vi "SDCP SMF Receiver and Transmitter - Test with plot.vi"() -> ()   [LabVIEW 2020]
uses:
  Typedefs/SDCP - Serial Port Control - Commands.ctl
  Typedefs/SDCP - Standard Message Frame Parameters - FGV - commands.ctl
  <vilib>/Utility/miscctls.llb/LVComboBoxStrsAndValuesArrayTypeDef.ctl
panel:
  in  "Remove frame":bool
  in  "Frame to add":string(combo)
  in  "Add frame":bool
  in  "Transmit Table":string[][](table)
  out "Elapsed time (ms)":u32
  in  "Parameter file path":path
  in  "Receive Table":i32(listbox)
  in  "stop":bool
  in  "VISA resource name":refnum<visa-resource-name>
  in  "Baud rate":u32=9600
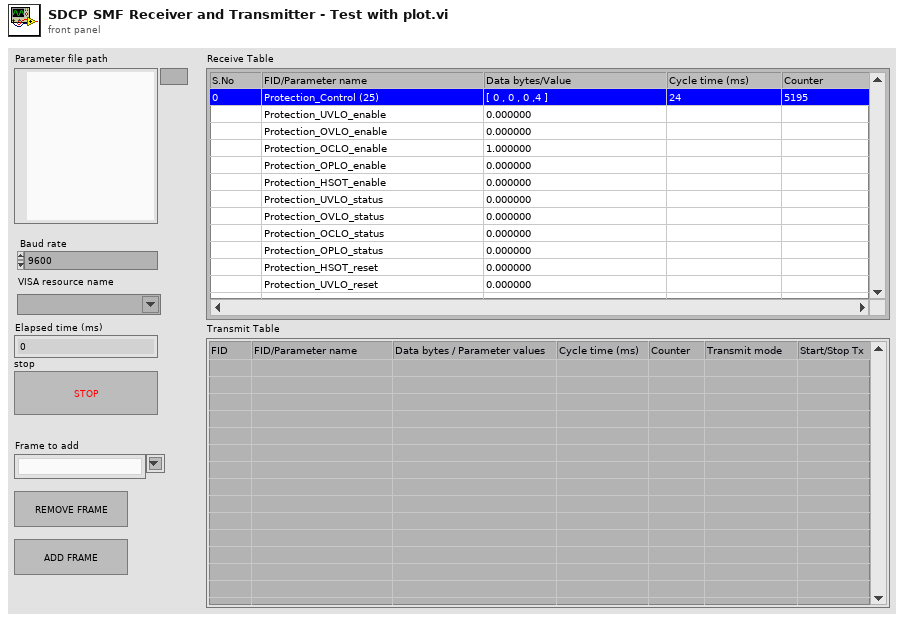
[diagram p1: front panel]
types:
  T1 = enum16{"Initialize", "Add row", "Remove row", "Update"}
  T2 = typedef "LVComboBoxStrsAndValuesArrayTypeDef.ctl" = cluster{"String":string, "Value":string}[]
  T3 = typedef "SDCP - Standard Message Frame Parameters - FGV - commands.ctl" = enum16{"Write descriptors", "Read descriptors", "Read values", "Load parameters from file", "Write values"}
  T4 = typedef "SDCP - Serial Port Control - Commands.ctl" = enum16{"Open", "Read", "Write", "Get instance", "Close"}
  T5 = typedef "SDCP - SMF parameter descriptors.ctl" = cluster{"Frame name":string, "Frame ID":i32, "Data type":string, "Start Position":i32, "Length":i32, "Factor":dbl, "Offset":dbl, "Parameter name":string, "Value":string}
  T6 = typedef "SDCP SMF Receiver and Transmitter - Notifier and Queues.ctl" = cluster{"Trace Queue":refnum<queue>, "Tx - Log Table Queue":refnum<queue>, "Tx - User Queue":refnum<queue>, "Rx - Log Table Queue":refnum<queue>, "Rx - User Queue":refnum<queue>, "Log status Notifier":refnum<notifier>, "Plot Queue":refnum<queue>}
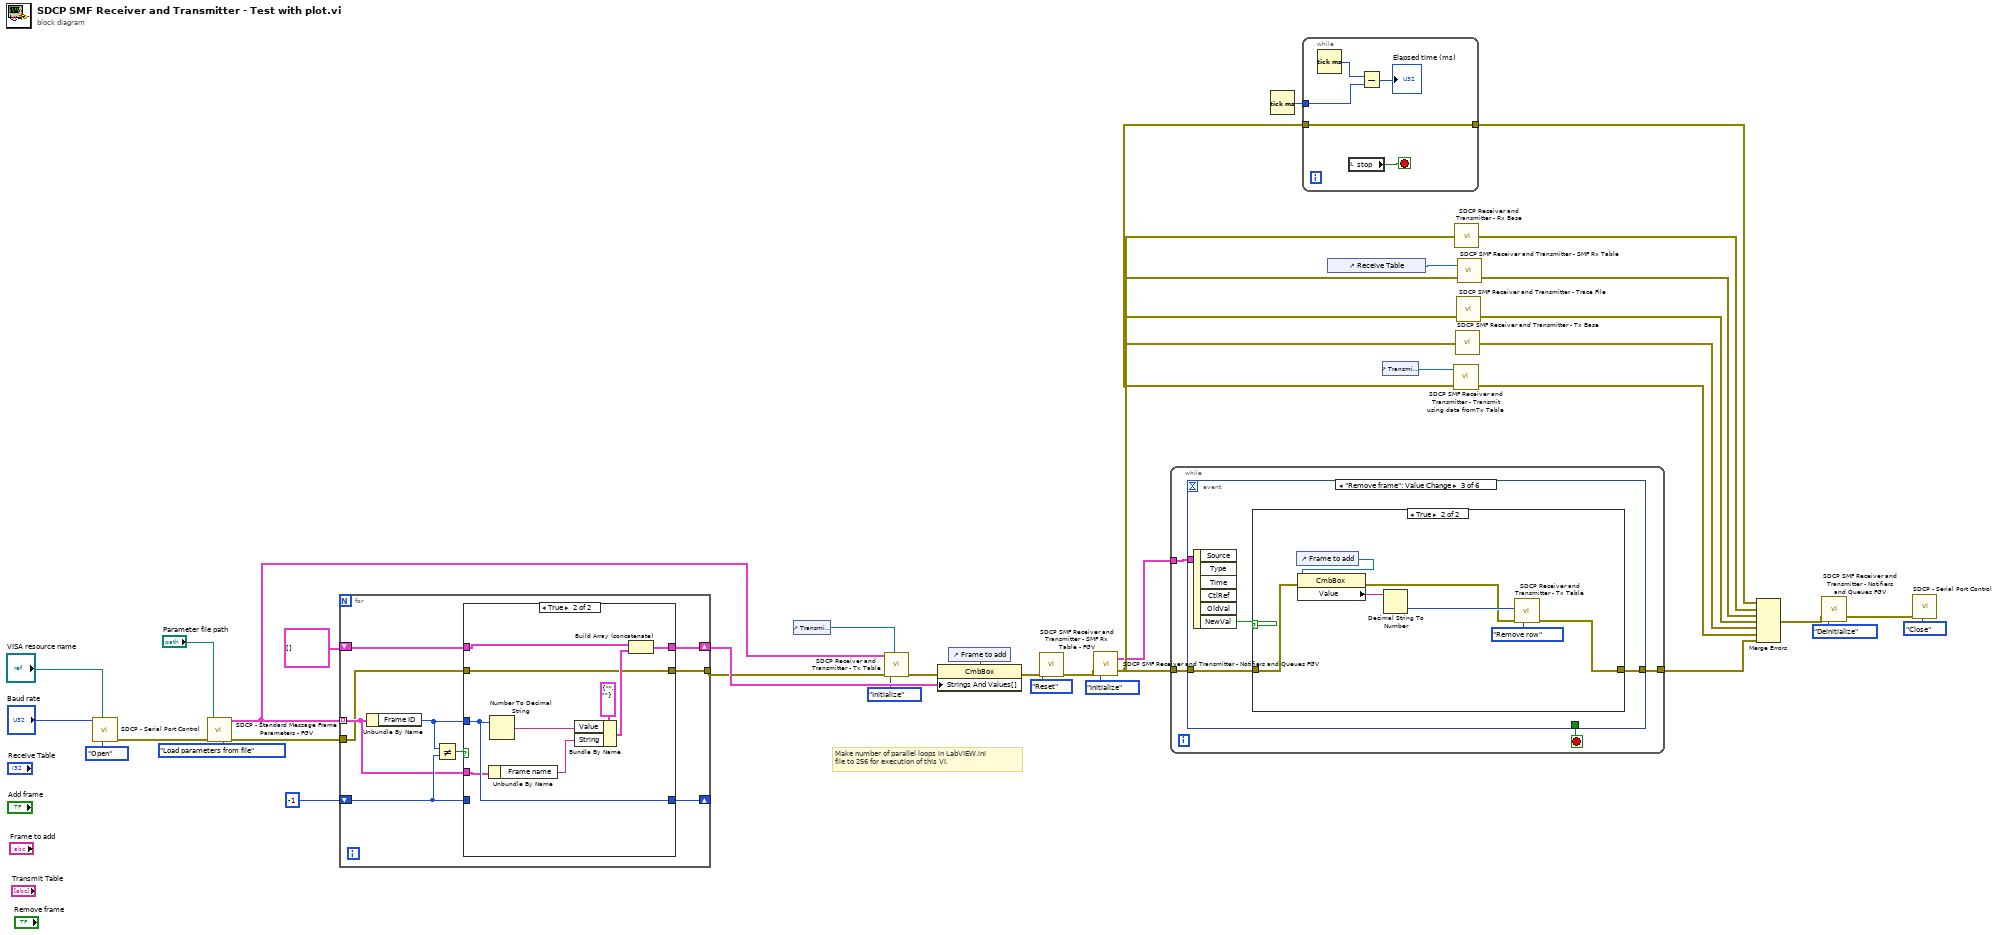
[diagram p0: block diagram]
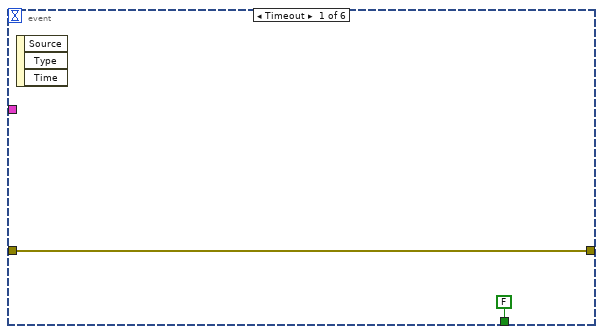
[diagram p2: hidden frame]
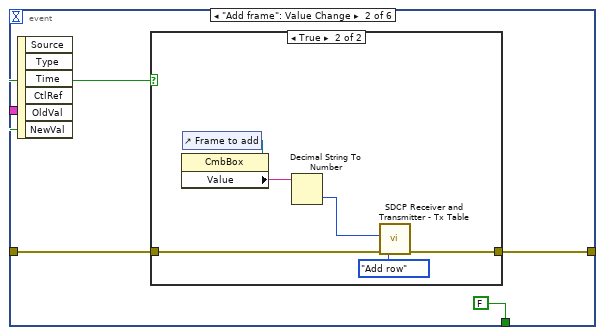
[diagram p3: hidden frame]
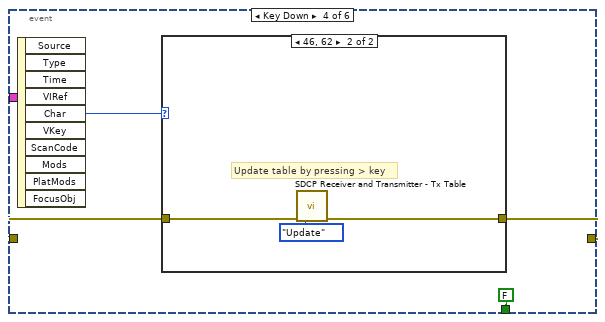
[diagram p6: hidden frame]
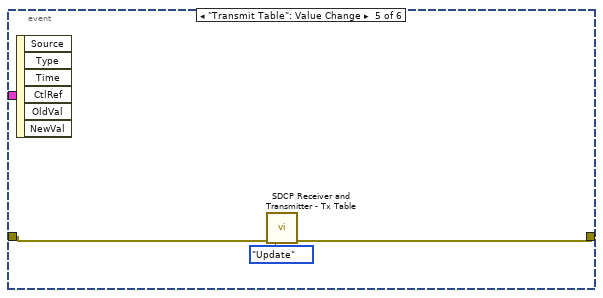
[diagram p8: hidden frame]
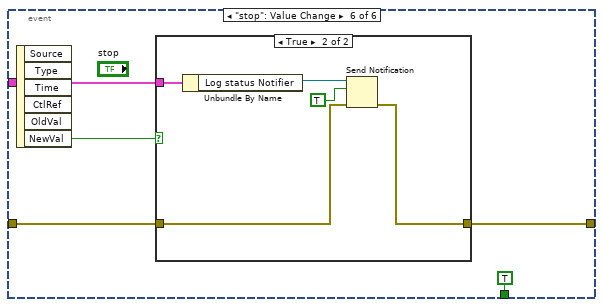
[diagram p9: hidden frame]
diagram:
  # "Make number of parallel loops in LabVIEW.ini\nfile to 256 for execution of this VI."
  n1 = call "SDCP - Serial Port Control.vi"("Command"=SDCP_-_Serial_Port_Control_-_Commands."Open", "VISA resource name"="VISA resource name", "Baud rate"="Baud rate") -> ("error out"=w22:errorcluster)  [unwired: 6 in, 2 out]
  n2 = call "SDCP - Standard Message Frame Parameters - FGV.vi"("Parameter file path"="Parameter file path", "error in (no error)"=w22, "Command"=SDCP_-_Standard_Message_Frame_Parameters_-_FGV_-_commands."Load parameters from file") -> ("SMF Parameters descriptors out"=w12:T5[], "error out"=w18:errorcluster)  [unwired: 4 in]
  n3 = for {
    tunnel: w18 -> [w38]
    tunnel: w12 -> [w39] mode=indexing
    shift-right: [w43] -> _
    shift-left: -1 -> [w42]
    shift-right: [w40] -> w14
    shift-left: T2 [] ("Strings And Values []") -> [w41]
    tunnel: [w37] -> w13
    n4 = Unbundle By Name(w39) -> ("Frame ID"=w44:i32)
    n5 = Not Equal?(x=w44, y=w42) -> (x != y?=w45:bool)
    n6 = case shown="True" w45 {
      tunnel: w44 -> [_ w57]
      tunnel: [w48 w57] -> w43
      tunnel: w42 -> [w48 _]
      tunnel: w41 -> [w47 w52]
      tunnel: [w47 w50] -> w40
      tunnel: w39 -> [_ w54]
      tunnel: w38 -> [w46 w49]
      tunnel: [w46 w49] -> w37
      frame False {
      }
      frame True {
        n7 = Unbundle By Name(w54) -> ("Frame name"=w53:string)
        n8 = Number To Decimal String(number=w57) -> (decimal integer string=w55:string)  [unwired: 1 in]
        n9 = Bundle By Name(cluster=cluster{"String":string, "Value":string} {"String"="", "Value"=""}, "Value"=w55, "String"=w53) -> (w51:cluster{"String":string, "Value":string})
        n10 = Build Array (concatenate)(w52, w51) -> (w50:T2)
      }
    }
  }
  n11 = control-ref of="Transmit Table"() -> (w9:refnum<vi>)
  n12 = call "SDCP Receiver and Transmitter - Tx Table.vi"("Table Control"=w9, "error in (no error)"=w13, "Command"=T1."Initialize", "SMF Parameters descriptors"=w12) -> ("error out"=w7:errorcluster)  [unwired: 6 in, 1 out]
  n13 = control-ref of="Frame to add"() -> (w8:refnum<vi>)
  n14 = property class="CmbBox"(reference=w8, error in=w7, "Strings And Values[]"=w14) -> (error out=w15:errorcluster)  [unwired: 1 out]
  n15 = call "SDCP SMF Receiver and Transmitter - SMF Rx Table - FGV.vi"("error in (no error)"=w15, "Command"=enum16{"Reset", "Write", "Read"}."Reset") -> ("error out"=w29:errorcluster)  [unwired: 8 in, 1 out]
  n16 = call "SDCP SMF Receiver and Transmitter - Notifiers and Queues FGV.vi"("error in (no error)"=w29, "Command"=enum16{"Initialize", "Read", "Deinitialize"}."Initialize") -> ("error out"=w5:errorcluster, "Output"=w1:T6)
  n17 = while {
    tunnel: w5 -> [w61]
    tunnel: [w60] -> w2
    tunnel: w1 -> [w58]
    stop <- w59 stop-if-true
    n18 = event shown="[2] \"Remove frame\": Value Change" {
      selector: _ -> [_ _ _ _ _ _]
      dyn-events: _ -> [_ _ _ _ _ _]
      timeout: _ -> [_ _ _ _ _ _]
      tunnel: w61 -> [w63 w66 w77 w88 w95 w98]
      tunnel: [w63 w65 w76 w87 w94 w97] -> w60
      tunnel: [FALSE FALSE _ FALSE _ TRUE] -> w59
      tunnel: w58 -> [_ _ _ _ _ w100]
      event Timeout {
        n19 = event-data() -> ()  [unwired: 1 in, 3 out]
      }
      event "Add frame": Value Change {
        n20 = event-data() -> ("NewVal"=w67:bool)  [unwired: 1 in, 5 out]
        n21 = case shown="True" w67 {
          tunnel: w66 -> [w68 w72]
          tunnel: [w68 w70] -> w65
          frame False {
          }
          frame True {
            n22 = control-ref of="Frame to add"() -> (w74:refnum<vi>)
            n23 = property class="CmbBox"(reference=w74) -> ("Value"=w73:string)  [unwired: 1 in, 2 out]
            n24 = Decimal String To Number(string=w73) -> (number=w71:i32)  [unwired: 2 in, 1 out]
            n25 = call "SDCP Receiver and Transmitter - Tx Table.vi"("error in (no error)"=w72, "Command"=T1."Add row", "FID"=w71) -> ("error out"=w70:errorcluster)  [unwired: 7 in, 1 out]
          }
        }
      }
      event "Remove frame": Value Change {
        n26 = event-data() -> ("NewVal"=w75:bool)  [unwired: 1 in, 5 out]
        n27 = case shown="True" w75 {
          tunnel: w77 -> [w78 w83]
          tunnel: [w78 w80] -> w76
          frame False {
          }
          frame True {
            n28 = control-ref of="Frame to add"() -> (w82:refnum<vi>)
            n29 = property class="CmbBox"(reference=w82, error in=w83) -> (error out=w81:errorcluster, "Value"=w85:string)  [unwired: 1 out]
            n30 = Decimal String To Number(string=w85) -> (number=w84:i32)  [unwired: 2 in, 1 out]
            n31 = call "SDCP Receiver and Transmitter - Tx Table.vi"("error in (no error)"=w81, "Command"=T1."Remove row", "FID"=w84) -> ("error out"=w80:errorcluster)  [unwired: 7 in, 1 out]
          }
        }
      }
      event Key Down {
        n32 = event-data() -> ("Char"=w86:i16)  [unwired: 1 in, 9 out]
        n33 = case shown="46, 62" w86 {
          tunnel: w88 -> [w90 w92]
          tunnel: [w90 w91] -> w87
          frame 0, Default {
          }
          frame 46, 62 {
            # "Update table by pressing > key"
            n34 = call "SDCP Receiver and Transmitter - Tx Table.vi"("error in (no error)"=w92, "Command"=T1."Update") -> ("error out"=w91:errorcluster)  [unwired: 8 in, 1 out]
          }
        }
      }
      event "Transmit Table": Value Change {
        n35 = event-data() -> ()  [unwired: 1 in, 6 out]
        n36 = call "SDCP Receiver and Transmitter - Tx Table.vi"("error in (no error)"=w95, "Command"=T1."Update") -> ("error out"=w94:errorcluster)  [unwired: 8 in, 1 out]
      }
      event "stop": Value Change {
        n37 = event-data() -> ("NewVal"=w99:bool)  [unwired: 1 in, 5 out]
        n38 = case shown="True" w99 {
          tunnel: w100 -> [_ w107]
          tunnel: w98 -> [w102 w104]
          tunnel: [w102 w103] -> w97
          frame False {
          }
          frame True {
            n39 = Unbundle By Name(w107) -> ("Log status Notifier"=w106:refnum<notifier>)
            n40 = Send Notification(notification=TRUE, notifier=w106, error in (no error)=w104) -> (error out=w103:errorcluster)  [unwired: 1 out]
          }
        }
      }
    }
  }
  n41 = Tick Count (ms)() -> (millisecond timer value=w19:u32)
  n42 = while {
    tunnel: w5 -> [w111]
    tunnel: [w111] -> w20
    tunnel: w19 -> [w109]
    stop <- w112 stop-if-true
    n43 = Tick Count (ms)() -> (millisecond timer value=w110:u32)
    n44 = local read "stop"() -> (w112:bool)
    n45 = Subtract(x=w110, y=w109) -> (x-y=→"Elapsed time (ms)":u32)
  }
  n46 = control-ref of="Receive Table"() -> (w27:refnum<vi>)
  n47 = control-ref of="Transmit Table"() -> (w6:refnum<vi>)
  n48 = call "SDCP SMF Receiver and Transmitter - Transmit using data fromTx Table.vi"("error in (no error)"=w5, "Table Control"=w6) -> ("error out"=w3:errorcluster)  [unwired: 3 in]
  n49 = call "SDCP Receiver and Transmitter - Rx Base.vi"("error in (no error)"=w5) -> ("error out"=w26:errorcluster)
  n50 = call "SDCP SMF Receiver and Transmitter - Tx Base.vi"("error in (no error)"=w5) -> ("error out"=w4:errorcluster)
  n51 = call "SDCP SMF Receiver and Transmitter - Trace File.vi"("error in (no error)"=w5) -> ("error out"=w21:errorcluster)  [unwired: 2 in]
  n52 = call "SDCP SMF Receiver and Transmitter - SMF Rx Table.vi"("error in (no error)"=w5, "Table reference"=w27) -> ("error out"=w25:errorcluster)  [unwired: 1 in]
  n53 = Merge Errors(w20, w26, w25, w21, w4, w3, w2) -> (w11:errorcluster)
  n54 = call "SDCP SMF Receiver and Transmitter - Notifiers and Queues FGV.vi"("error in (no error)"=w11, "Command"=enum16{"Initialize", "Read", "Deinitialize"}."Deinitialize") -> ("error out"=w31:errorcluster)  [unwired: 1 out]
  n55 = call "SDCP - Serial Port Control.vi"("Command"=SDCP_-_Serial_Port_Control_-_Commands."Close", "error in (no error)"=w31) -> ()  [unwired: 7 in, 3 out]
